vi "pump fpga.vi"() -> ()   [LabVIEW 2017]
uses:
  <vilib>/rvi/Emulation/niFpgaGetClockAttributes.vi
  <vilib>/rvi/Emulation/niFpgaSctlEmulationGetInTimedLoop.vi
  <vilib>/rvi/Emulation/niFpgaEmulationReportErrorSimple.vi
  <vilib>/rvi/eio/common/nirviEmuTemplateMethod_errors.vi
  <vilib>/rvi/Emulation/niFpgaCriticalErrorInLSC.vi
  <vilib>/eio/EIONode/EIONode.xnode
panel:
  out "ConnectorB/DIO4":bool
  out "ConnectorB/DIO3":bool
  out "ConnectorB/DIO2":bool
  out "ConnectorB/DIO1":bool
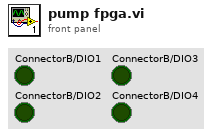
[diagram p1: front panel]
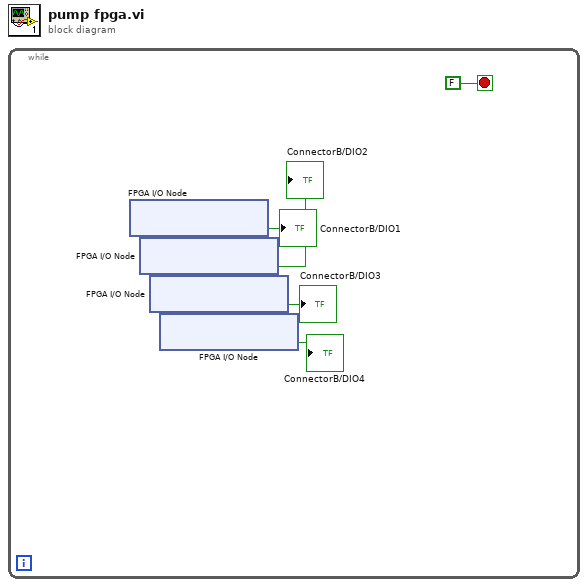
[diagram p0: block diagram]
diagram:
  n1 = while {
    stop <- FALSE stop-if-true
    n2 = xnode "FPGA I/O Node"() -> ("ConnectorC/DIO3"=→"ConnectorB/DIO1":bool)  [unwired: 1 in, 1 out]
    n3 = xnode "FPGA I/O Node"() -> ("ConnectorC/DIO4"=→"ConnectorB/DIO2":bool)  [unwired: 1 in, 1 out]
    n4 = xnode "FPGA I/O Node"() -> ("ConnectorC/DIO5"=→"ConnectorB/DIO3":bool)  [unwired: 1 in, 1 out]
    n5 = xnode "FPGA I/O Node"() -> ("ConnectorC/DIO6"=→"ConnectorB/DIO4":bool)  [unwired: 1 in, 1 out]
  }
